vi "DMM_Scan PMPS 16V-15C Close.vi"(0 "Scan Resources Handles In":T1, 11 "error in":errorcluster) -> (15 "error out":errorcluster)   [LabVIEW 2021, in "DMM_Scan PXI Mux PXI Shunt 16V-15C.lvlib"]
doc: "Disconnects all Multiplexer and Shunt Relays and closes the NI-DMM and NI SWITCH Scan session specifed in Scan Resources Handle In and releases all resources."
uses:
  DMM_Scan PXI Mux PXI Shunt 16V-15C.lvlib
  Typedefs/Scan Resource Handles In.ctl
  DMM Mixed Measurements/DMM_Mixed Measurement.lvlib
  Static Digital Path Generation/Switch_Static Digital Path Generation.lvlib
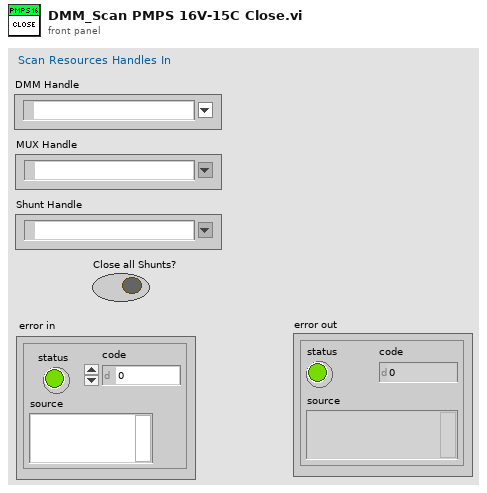
[diagram p1: front panel]
types:
  T1 = typedef "DMM_Scan PXI Mux PXI Shunt 16V-15C.lvlib/Scan Resource Handles In.ctl" = cluster{"DMM Handle":refnum<k15>, "MUX Handle":refnum<k15>, "Shunt Handle":refnum<k15>, "Close all Shunts?":bool}
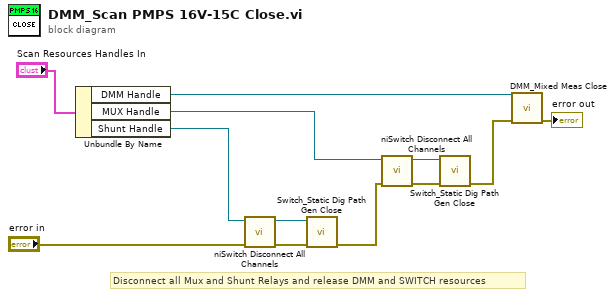
[diagram p0: block diagram]
diagram:
  # "Disconnect all Mux and Shunt Relays and release DMM and SWITCH resources"
  n1 = Unbundle By Name("Scan Resources Handles In") -> ("DMM Handle"=w10:refnum<k15>, "MUX Handle"=w4:refnum<k15>, "Shunt Handle"=w6:refnum<k15>)
  n2 = call <instrlib>:"niSwitch Disconnect All Channels.vi"("error in (no error)"="error in", "instrument handle"=w6) -> ("error out"=w8:errorcluster, "instrument handle out"=w7:refnum<k15>)  [unwired: 8 in]
  n3 = call "Switch_Static Dig Path Gen Close.vi"("Switch Handle In"=w7, "error in"=w8) -> ("error out"=w1:errorcluster)  [unwired: 13 in]
  n4 = call <instrlib>:"niSwitch Disconnect All Channels.vi"("error in (no error)"=w1, "instrument handle"=w4) -> ("error out"=w2:errorcluster, "instrument handle out"=w3:refnum<k15>)  [unwired: 8 in]
  n5 = call "Switch_Static Dig Path Gen Close.vi"("Switch Handle In"=w3, "error in"=w2) -> ("error out"=w11:errorcluster)  [unwired: 13 in]
  n6 = call "DMM_Mixed Meas Close.vi"("DMM Handle In"=w10, "error in"=w11) -> ("error out"=→"error out":errorcluster)  [unwired: 13 in]
